vi "Common_TempCangeLabelName.vi"(1 "Path":path, 2 "String":string) -> (15 "PathOut":path)   [LabVIEW 2020]
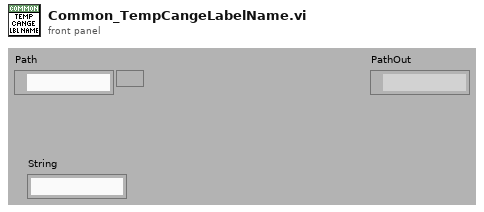
[diagram p1: front panel]
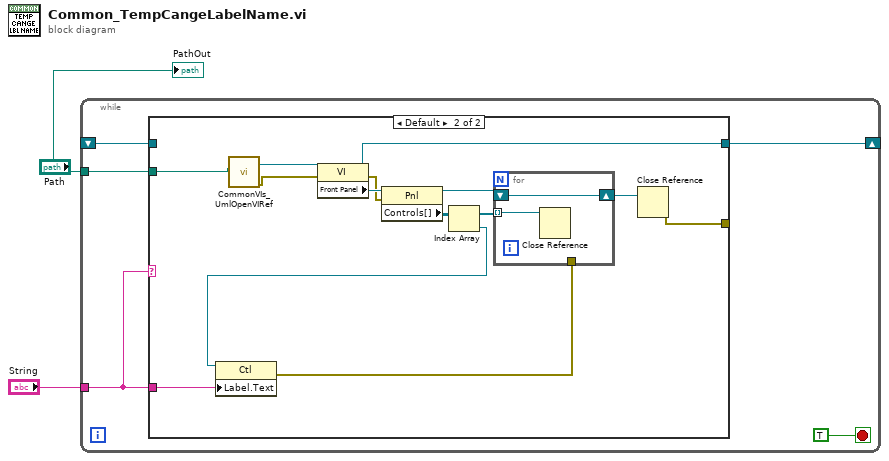
[diagram p0: block diagram]
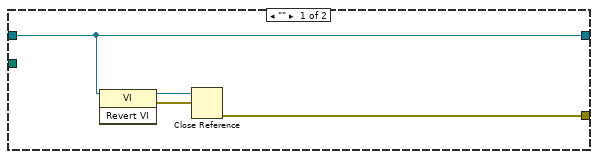
[diagram p2: hidden frame]
diagram:
  n1 = while {
    tunnel: "Path" -> [w7]
    tunnel: "String" -> [w6]
    shift-right: [w4] -> _
    shift-left: _ -> [w3]
    stop <- TRUE stop-if-true
    n2 = case shown="Default" w6 {
      tunnel: w7 -> [_ w15]
      tunnel: w6 -> [_ w19]
      tunnel: [w11 w17] -> w4
      tunnel: w3 -> [w11 _]
      tunnel: [w8 w12] -> _
      frame "" {
        n3 = invoke class="VI" method="Revert VI"(reference=w11) -> (reference out=w10:refnum<vi>, error out=w9:errorcluster)  [unwired: 2 in, 1 out]
        n4 = Close Reference(reference=w10, error in (no error)=w9) -> (error out=w8:errorcluster)
      }
      frame Default {
        n5 = call <resource>:"CommonVIs_UmlOpenVIRef.vi"("ViPath/ViName"=w15) -> ("error out"=w13:errorcluster, "vi reference"=w14:refnum<vi>)  [unwired: 3 in, 6 out]
        n6 = property class="VI"(reference=w14, error in=w13) -> (reference out=w17:refnum<vi>, error out=w23:errorcluster, "Front Panel"=w24:refnum<vi>)
        n7 = property class="Pnl"(reference=w24, error in=w23) -> (reference out=w21:refnum<vi>, "Controls[]"=w22:refnum<vi>[])  [unwired: 1 out]
        n8 = Index Array(array=w22) -> (element=w20:refnum<vi>)  [unwired: 1 in]
        n9 = property class="Ctl"(reference=w20, "Label.Text"=w19) -> (error out=w18:errorcluster)  [unwired: 1 in, 1 out]
        n10 = for {
          tunnel: w22 -> [w26] mode=indexing
          shift-right: [w25] -> w16
          shift-left: w21 -> [w25]
          tunnel: w18 -> [_]
          n11 = Close Reference(reference=w26) -> ()  [unwired: 1 in, 1 out]
        }
        n12 = Close Reference(reference=w16) -> (error out=w12:errorcluster)  [unwired: 1 in]
      }
    }
  }
  "PathOut" <- "Path"
